vi "ScriptOneofClassConverter.vi"(8 "error in (no error)":errorcluster, 9 "Generate_SerializationHelper":bool, 10 "Oneof container name":string, 11 "Library":refnum<vi>) -> (0 "error out":errorcluster, 3 "Library out":refnum<vi>)   [LabVIEW 2019, in "gRPC Template Creation Utility.lvlib"]
uses:
  gRPC Template Creation Utility.lvlib
  <vilib>/Utility/traverseref.llb/TRef TravTarget.ctl
  <vilib>/Utility/traverseref.llb/VI Scripting - Traverse.lvlib
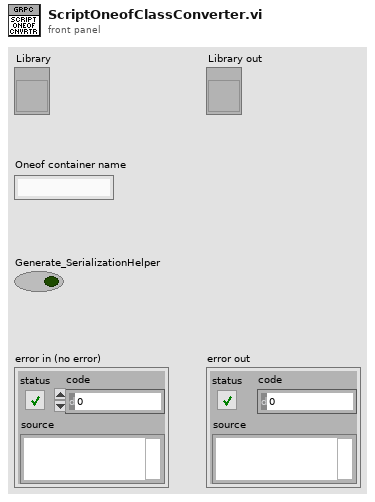
[diagram p1: front panel]
types:
  T1 = typedef "TRef TravTarget.ctl" = enum16{"FP", "BD", "Other"}
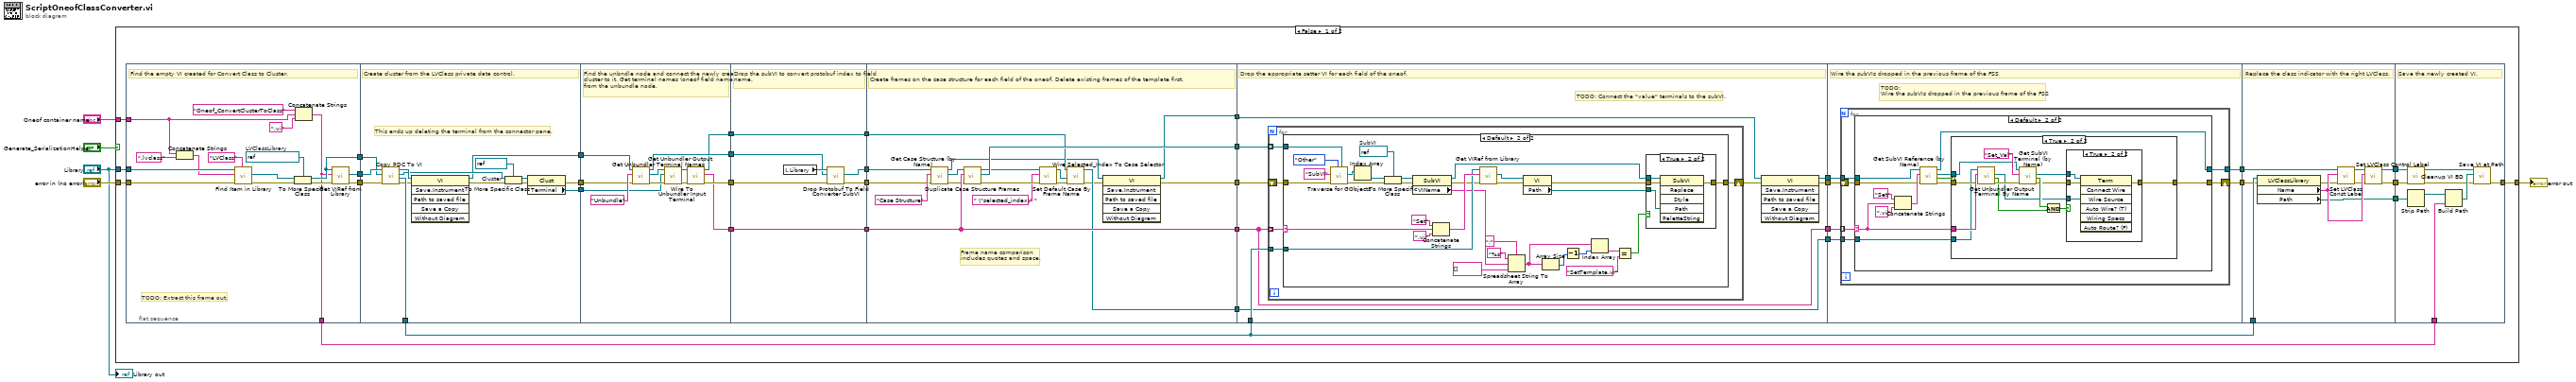
[diagram p0: block diagram]
diagram:
  n1 = case shown="False" "Generate_SerializationHelper" {
    tunnel: "error in (no error)" -> [w39 w223]
    tunnel: [w35 w223] -> w4
    tunnel: "Library" -> [w27 _]
    tunnel: "Oneof container name" -> [w25 _]
    frame False {
      n2 = flat-sequence {
        tunnel: w39 -> [w46]
        tunnel: [w55] -> w30
        tunnel: [w44] -> w29
        tunnel: [w54] -> w28
        tunnel: w27 -> [w51]
        tunnel: [w40] -> w26
        tunnel: w25 -> [w41]
        tunnel: [w66] -> w36
        tunnel: [w60] -> w24
        tunnel: [w57] -> w23
        tunnel: w30 -> [w69]
        tunnel: w29 -> [w68]
        tunnel: w28 -> [w65]
        tunnel: [w61] -> w22
        tunnel: w24 -> [w78]
        tunnel: w23 -> [w76]
        tunnel: [w71] -> w21
        tunnel: [w81] -> w19
        tunnel: [w74] -> w17
        tunnel: w22 -> [w72]
        tunnel: [w70] -> w12
        tunnel: w21 -> [w88]
        tunnel: [w88] -> w20
        tunnel: w19 -> [w82]
        tunnel: [w87] -> w18
        tunnel: w17 -> [w85]
        tunnel: [w83] -> w16
        tunnel: w12 -> [w84]
        tunnel: [w84] -> w11
        tunnel: w20 -> [w106]
        tunnel: w18 -> [w101]
        tunnel: w16 -> [w103]
        tunnel: [w106] -> w38
        tunnel: [w105] -> w37
        tunnel: [w89] -> w32
        tunnel: w11 -> [w98]
        tunnel: [w95] -> w10
        tunnel: [w99] -> w7
        tunnel: w38 -> [w113]
        tunnel: w37 -> [w111]
        tunnel: w36 -> [w114]
        tunnel: [w108] -> w15
        tunnel: w32 -> [w110]
        tunnel: w10 -> [w115]
        tunnel: [w113] -> w9
        tunnel: [w112] -> w8
        tunnel: w7 -> [w112]
        tunnel: [w107] -> w6
        tunnel: w15 -> [w164]
        tunnel: [w161] -> w14
        tunnel: [w162] -> w13
        tunnel: w9 -> [w163]
        tunnel: w8 -> [w160]
        tunnel: w6 -> [w159]
        tunnel: w14 -> [w209]
        tunnel: w36 -> [w212]
        tunnel: [w205] -> w34
        tunnel: [w204] -> w33
        tunnel: w13 -> [w213]
        tunnel: [w210] -> w31
        tunnel: [w219] -> w35
        tunnel: w34 -> [w216]
        tunnel: w33 -> [w218]
        tunnel: w31 -> [w222]
        tunnel: w26 -> [w215]
        frame #0 {
          w48 = refnum<vi> refnum  # LVClassLibrary
          # "TODO: Extract this frame out."
          # "Find the empty VI created for Convert Class to Cluster."
          n3 = Concatenate Strings(w41, ".lvclass" ("string")) -> (w43:string)
          n4 = call "Find Item in Library.vi"("Item Type"="LVClass", "error in (no error)"=w46, "Item Name"=w43, "Library item in"=w51) -> ("error out"=w47:errorcluster, "Project Item (Library Item)"=w49:refnum<vi>)  [unwired: 4 in, 2 out]
          n5 = To More Specific Class(target class=w48, reference=w49, error in=w47) -> (specific class reference=w44:refnum<vi>, error out=w45:errorcluster)
          n6 = Concatenate Strings("Oneof_ConvertClusterToClass" ("format string"), w41, ".vi" ("string")) -> (w40:string)
          n7 = call "Get VIRef from Library.vi"("error in (no error)"=w45, "item name"=w40, "library in"=w44) -> ("error out"=w54:errorcluster, "vi"=w55:refnum<vi>)  [unwired: 5 in, 2 out]
        }
        frame #1 {
          w63 = refnum<vi> refnum  # Cluster
          # "This ends up deleting the terminal from the connector pane."
          # "Create cluster from the LVClass private data control."
          n8 = call "Copy PDC To VI.vi"("error in (no error)"=w65, "LVClassLibrary Refnum in"=w68, "VI in"=w69) -> ("error out"=w58:errorcluster, "LVClassLibrary Refnum out"=w66:refnum<vi>, "Cluster Ref"=w64:refnum<vi>, "VI out"=w67:refnum<vi>)  [unwired: 5 in]
          n9 = invoke class="VI" method="Save.Instrument"(reference=w67, error in=w58) -> (reference out=w60:refnum<vi>, error out=w59:errorcluster)  [unwired: 4 in, 4 out]
          n10 = To More Specific Class(target class=w63, reference=w64, error in=w59) -> (specific class reference=w62:refnum<vi>, error out=w56:errorcluster)
          n11 = property class="Clust"(reference=w62, error in=w56) -> (error out=w57:errorcluster, "Terminal"=w61:refnum<vi>)  [unwired: 1 out]
        }
        frame #2 {
          # "Find the unbndle node and connect the newly created cluster to it. Get terminal names (oneof field names) from the unbundle node."
          n12 = call "Get Unbundler.vi"("error in (no error)"=w76, "Label"="Unbundle" ("Class Name"), "Owner VI in"=w78) -> ("error out"=w73:errorcluster, "Unbundler Refnum"=w75:refnum<vi>, "Owner VI out"=w74:refnum<vi>)  [unwired: 5 in, 1 out]
          n13 = call "Wire To Unbundler Input Terminal.vi"("error in (no error)"=w73, "Terminal to be wired"=w72, "Unbundler in"=w75) -> ("error out"=w79:errorcluster, "Unbundler out"=w80:refnum<vi>)  [unwired: 7 in]
          n14 = call "Get Unbundler Output Terminal Names.vi"("error in (no error)"=w79, "Unbundler in"=w80) -> ("error out"=w81:errorcluster, "Terminal names"=w71:string[], "Unbundler out"=w70:refnum<vi>)  [unwired: 7 in]
        }
        frame #3 {
          # "Drop the subVI to convert protobuf index to field name."
          n15 = local read "Library"() -> (w86:refnum<vi>)
          n16 = call "Drop Protobuf To Field Converter SubVI.vi"("error in (no error)"=w82, "Owner VI in"=w85, "Library"=w86) -> ("error out"=w87:errorcluster, "Owner VI out"=w83:refnum<vi>)  [unwired: 5 in, 2 out]
        }
        frame #4 {
          # "Frame name comparison\nincludes quotes and space."
          # "Create frames on the case structure for each field of the oneof. Delete existing frames of the template first."
          n17 = call "Get Case Structure (by Name).vi"("error in (no error)"=w101, "Case Structure name"="Case Structure" ("Class Name"), "VI ref in"=w103) -> ("error out"=w104:errorcluster, "CaseStructure out"=w100:refnum<vi>, "VI ref out"=w97:refnum<vi>)  [unwired: 5 in, 1 out]
          n18 = call "Duplicate Case Structure Frames.vi"("error in (no error)"=w104, "Frame Names"=w106, "CaseStructure in"=w100) -> ("error out"=w94:errorcluster, "Case Frames[]"=w105:refnum<vi>[], "CaseStructure out"=w93:refnum<vi>)  [unwired: 6 in]
          n19 = call "Set Default Case By Frame Name.vi"("error in (no error)"=w94, "Frame Name"=" \"selected_index\" ", "CaseStructure in"=w93) -> ("error out"=w91:errorcluster, "CaseStructure out"=w92:refnum<vi>)  [unwired: 7 in]
          n20 = call "Wire Selected_Index To Case Selector.vi"("error in (no error)"=w91, "CaseStructure in"=w92, "Unbundler in"=w98) -> ("error out"=w96:errorcluster, "Unbundler out"=w99:refnum<vi>)  [unwired: 5 in, 2 out]
          n21 = invoke class="VI" method="Save.Instrument"(reference=w97, error in=w96) -> (reference out=w89:refnum<vi>, error out=w95:errorcluster)  [unwired: 4 in, 4 out]
        }
        frame #5 {
          # "TODO: Connect the \"value\" terminals to the subVI."
          # "Drop the appropriate setter VI for each field of the oneof."
          n22 = for {
            tunnel: w111 -> [w120] mode=indexing
            tunnel: w113 -> [w117] mode=indexing
            shift-right: [w116] -> w109
            shift-left: w115 -> [w119]
            tunnel: w114 -> [w118]
            n23 = case shown="Default" w117 {
              selector: w117 -> [_ w147]
              tunnel: w120 -> [_ w132]
              tunnel: w119 -> [w121 w144]
              tunnel: [w121 w136] -> w116
              tunnel: w118 -> [_ w148]
              frame "selected_index" {
                # "Do nothing."
              }
              frame Default {
                w141 = refnum<vi> refnum  # SubVI
                n24 = call <vilib>:"Traverse for GObjects.vi"("Other Refnum"=w132, "Traverse Target"=TRef_TravTarget."Other", "error in (no error)"=w144, "Class Name"="SubVI") -> ("error out"=w134:errorcluster, "References"=w143:refnum<vi>[])  [unwired: 4 in, 2 out]
                n25 = Index Array(array=w143) -> (element=w142:refnum<vi>)  [unwired: 1 in]
                n26 = To More Specific Class(target class=w141, reference=w142, error in=w134) -> (specific class reference=w140:refnum<vi>, error out=w133:errorcluster)
                n27 = property class="SubVI"(reference=w140, error in=w133) -> (reference out=w139:refnum<vi>, error out=w135:errorcluster, "VIName"=w129:string)
                n28 = Concatenate Strings("Set" ("string"), w147, ".vi" ("string")) -> (w151:string)
                n29 = call "Get VIRef from Library.vi"("error in (no error)"=w135, "item name"=w151, "library in"=w148) -> ("error out"=w149:errorcluster, "vi"=w150:refnum<vi>)  [unwired: 5 in, 2 out]
                n30 = Spreadsheet String To Array(delimiter (Tab)=":", format string="%s", spreadsheet string=w129, array type (2D Dbl)=string[] []) -> (array=w125:string[])
                n31 = property class="VI"(reference=w150, error in=w149) -> (error out=w130:errorcluster, "Path"=w131:path)  [unwired: 1 out]
                n32 = Array Size(array=w125) -> (size(s)=w124:i32)
                n33 = Decrement(x=w124) -> (x-1=w123:i32)
                n34 = Index Array(array=w125, index=w123) -> (element=w122:string)
                n35 = Equal?(x=w122, y="SetTemplate.vi" ("string")) -> (x = y?=w137:bool)
                n36 = case shown="True" w137 {
                  tunnel: w139 -> [_ w158]
                  tunnel: [w154 w157] -> w136
                  tunnel: w131 -> [_ w156]
                  tunnel: w130 -> [w154 w155]
                  frame False {
                  }
                  frame True {
                    n37 = invoke class="SubVI" method="Replace"(reference=w158, error in=w155, "Path"=w156) -> (error out=w157:errorcluster)  [unwired: 3 in, 5 out]
                  }
                }
              }
            }
          }
          n38 = invoke class="VI" method="Save.Instrument"(reference=w110, error in=w109) -> (reference out=w107:refnum<vi>, error out=w108:errorcluster)  [unwired: 4 in, 4 out]
        }
        frame #6 {
          # "TODO:\nWire the subVIs dropped in the previous frame of the FSS"
          # "Wire the subVIs dropped in the previous frame of the FSS"
          n39 = for {
            tunnel: w163 -> [w169] mode=indexing
            shift-right: [w168] -> w161
            shift-left: w164 -> [w170]
            tunnel: w159 -> [w167]
            tunnel: [w166] -> w162
            tunnel: w160 -> [w165]
            n40 = case shown="Default" w169 {
              selector: w169 -> [_ w176]
              tunnel: w170 -> [w172 w179]
              tunnel: [w172 w173] -> w168
              tunnel: w167 -> [w171 w182]
              tunnel: [w171 w181] -> w166
              tunnel: w165 -> [_ w178]
              frame "selected_index" {
                # "Do nothing."
              }
              frame Default {
                n41 = Concatenate Strings("Set" ("string"), w176, ".vi" ("string")) -> (w183:string)
                n42 = call "Get SubVI Reference (by Name).vi"("error in (no error)"=w179, "SubVI Name"=w183, "Owner VI in"=w182) -> ("error out"=w174:errorcluster, "Found ?"=w177:bool, "SubVI Refnum out"=w175:refnum<vi>, "Owner VI out"=w181:refnum<vi>)  [unwired: 5 in]
                n43 = case shown="True" w177 {
                  tunnel: w175 -> [_ w195]
                  tunnel: w176 -> [_ w198]
                  tunnel: w174 -> [w185 w197]
                  tunnel: [w185 w187] -> w173
                  tunnel: w178 -> [_ w186]
                  frame False {
                  }
                  frame True {
                    n44 = call "Get Unbundler Output Terminal By Name.vi"("error in (no error)"=w197, "Terminal name"=w198, "Unbundler in"=w186) -> ("error out"=w194:errorcluster, "Found?"=w192:bool, "Terminal Refnum"=w190:refnum<vi>)  [unwired: 5 in, 1 out]
                    n45 = call "Get SubVI Terminal (by Name).vi"("error in (no error)"=w194, "Terminal name"="Set_Val", "SubVI in"=w195) -> ("error out"=w188:errorcluster, "Found?"=w191:bool, "SubVI Term ref"=w189:refnum<vi>)  [unwired: 5 in, 1 out]
                    n46 = And(x=w191, y=w192) -> (x .and. y?=w193:bool)
                    n47 = case shown="True" w193 {
                      tunnel: w190 -> [_ w202]
                      tunnel: w189 -> [_ w203]
                      tunnel: w188 -> [w199 w201]
                      tunnel: [w199 w200] -> w187
                      frame False {
                      }
                      frame True {
                        n48 = invoke class="Term" method="Connect Wire"(reference=w203, error in=w201, "Wire Source"=w202) -> (error out=w200:errorcluster)  [unwired: 4 in, 6 out]
                      }
                    }
                  }
                }
              }
            }
          }
        }
        frame #7 {
          # "Replace the class indicator with the right LVClass."
          n49 = property class="LVClassLibrary"(reference=w212, error in=w209) -> (error out=w207:errorcluster, "Name"=w211:string, "Path"=w210:path)  [unwired: 1 out]
          n50 = call "Set LVClass Const Label.vi"("error in (no error)"=w207, "Class name"=w211, "VI in"=w213) -> ("error out"=w206:errorcluster, "VI out"=w208:refnum<vi>)  [unwired: 7 in]
          n51 = call "Set LVClass Control Label.vi"("error in (no error)"=w206, "Name"=w211, "VI in"=w208) -> ("error out"=w205:errorcluster, "VI out"=w204:refnum<vi>)  [unwired: 7 in]
        }
        frame #8 {
          # "Save the newly created VI."
          n52 = call "Cleanup VI BD.vi"("error in (no error)"=w216, "VI in"=w218) -> ("error out"=w214:errorcluster, "VI out"=w217:refnum<vi>)  [unwired: 8 in]
          n53 = Strip Path(path=w222) -> (stripped path=w221:path)  [unwired: 1 out]
          n54 = Build Path(base path=w221, name or relative path=w215) -> (appended path=w220:path)
          n55 = call "Save VI at Path.vi"("error in (no error)"=w214, "Path"=w220, "VI in"=w217) -> ("error out"=w219:errorcluster)  [unwired: 6 in, 2 out]
        }
      }
    }
    frame True {
      # "If LVClass is an invalid refnum (the message probably doesn't have a oneof), then ignore it."
    }
  }
  "error out" <- w4
  "Library out" <- "Library"
